vi "19572 Get_test_TIME.vi"(8 "error in (no error)":errorcluster, 9 "Step":u16=1 min=1 max=99 step=1, 11 "VISA resource in":refnum<visa-resource-name>) -> (0 "error out":errorcluster, 1 "Test TIME":dbl format="%.1p", 3 "VISA resource out":refnum<visa-resource-name>)   [LabVIEW 2015]
panel:
  out "output command":string
  # "Get GB test TIME"
  # "[s]"
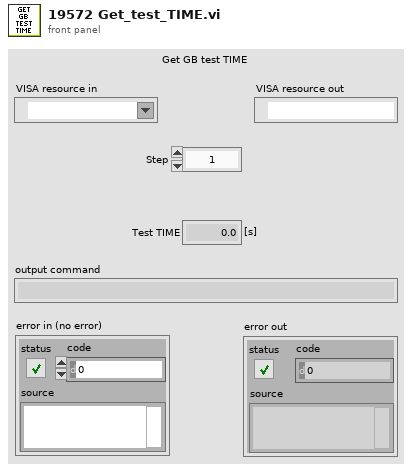
[diagram p1: front panel]
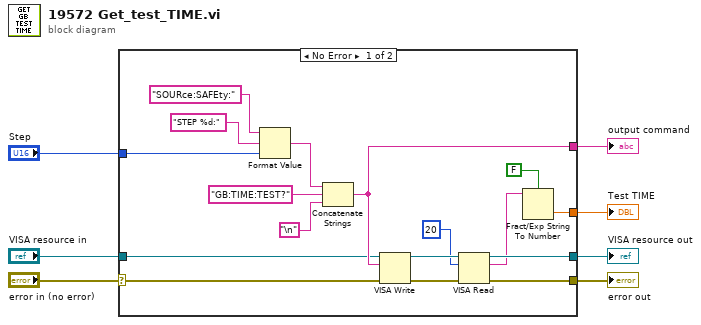
[diagram p0: block diagram]
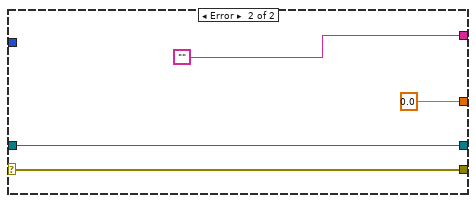
[diagram p2: hidden frame]
diagram:
  n1 = case shown="No Error" "error in (no error)" {
    selector: "error in (no error)" -> [w24 w28]
    tunnel: [w18 w28] -> w7
    tunnel: [w15 ""] -> w5
    tunnel: [w14 w26] -> w4
    tunnel: "Step" -> [w13 _]
    tunnel: "VISA resource in" -> [w12 w26]
    tunnel: [w10 0.0] -> w1
    frame No Error {
      n2 = Format Value(string ("")="SOURce:SAFEty:", format string="STEP %d:", value (0)=w13) -> (output string=w8:string)
      n3 = Concatenate Strings(w8, "GB:TIME:TEST?", "\n") -> (w15:string)
      n4 = VISA Write(VISA resource name=w12, write buffer=w15, error in (no error)=w24) -> (VISA resource name out=w17:refnum<visa-resource-name>, error out=w19:errorcluster)  [unwired: 1 out]
      n5 = VISA Read(VISA resource name=w17, byte count=u32 20, error in (no error)=w19) -> (VISA resource name out=w14:refnum<visa-resource-name>, read buffer=w11:string, error out=w18:errorcluster)  [unwired: 1 out]
      n6 = Fract/Exp String To Number(use system decimal point (T)=FALSE, string=w11) -> (number=w10:dbl)  [unwired: 2 in, 1 out]
    }
    frame Error {
    }
  }
  "error out" <- w7
  "VISA resource out" <- w4
  "output command" <- w5
  "Test TIME" <- w1
